vi "Set Value.vi"(9 "Value In":variant, 11 "Ref In":refnum<vi>) -> ()   [LabVIEW 2024]
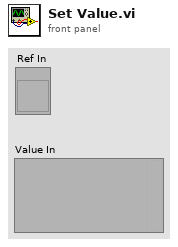
[diagram p1: front panel]
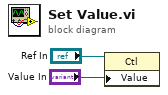
[diagram p0: block diagram]
diagram:
  n1 = property class="Ctl"(reference="Ref In", "Value"="Value In") -> ()  [unwired: 1 in, 2 out]
